vi "Main.vi"() -> ()   [LabVIEW 2020]
uses:
  Typedef/Product Installer.ctl
  Typedef/Custom Action.ctl
  Typedef/Product Installer Definition.ctl
  Typedef/Custom Action Definition.ctl
  Typedef/State.ctl
  Bundle Builder/Bundle Builder.lvclass
  Bundle Builder/Bundle Builder.lvclass/Bundle Builder.ctl
  bd79d48e-615b-41ab-9cb3-2d2f9496b7e1.vi
  Bundle Builder/Read Bundle Definition.vi
  Bundle Builder/Read Bundle Root.vi
  Bundle Builder/Read Product Installers.vi
  Bundle Builder/Read Custom Actions.vi
  Bundle Builder/Read Element of Custom Actions Defnition.vi/bd8829dc-8fc1-4ce8-8fca-fa4916f1d24d.vi
  Bundle Builder/Read Element of Product Installers Definition.vi/92f76918-1563-4c6f-99b4-6a0cba476cd6.vi
  <vilib>/Comparison/Equal/Equal Functor/Equal Functor.lvclass
panel:
  in  "New":bool
  in  "Clear Disk":bool
  in  "Stop Button":bool
  in  "Save":bool
  in  "Tab":T1(tab)
  out "Bundle Root Folder":path
  in  "Bundle Definition":T2
  out "Product Key Unique?":bool
  in  "Product Installers":T3[](array[typedef])
  in  "Product Installer":T4 caption="NI Product Installer / Custom Product Installer"
  in  "Custom Actions":T5[](array[typedef])
  out "Custom Action Key Unique?":bool
  in  "Custom Action":T6
  in  "Open":bool
  in  "Definitions":string(tree)
  # "STS Custom Bundle Builder"
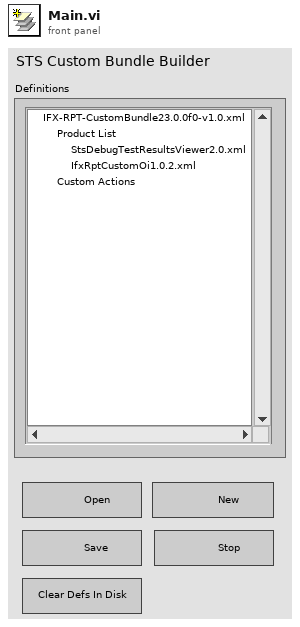
[diagram p1: front panel]
types:
  T1 = enum32{"Default", "Bundle", "Product List", "Product", "Custom Actions", "Custom Action"}
  T2 = cluster{"Key":string, "Display Name":string, "STS Software":string}
  T3 = typedef "Product Installer.ctl" = cluster{"Key":string, "Version":string, "Type":enum16{"NI Installer", "Custom Installer"}}
  T4 = typedef "Product Installer Definition.ctl" = cluster{"Display Name":string, "Install Commands":cluster{"Path":string, "Parameters":string, "Successful Exit Codes":string, "Log Command":cluster{"Flag":string, "File Name":string}}[], "Uninstall Commands":cluster{"Path":string, "Parameters":string, "Successful Exit Codes":string, "Log Command":cluster{"Flag":string, "File Name":string}}[]}
  T5 = typedef "Custom Action.ctl" = cluster{"Key":string, "Timing":string}
  T6 = typedef "Custom Action Definition.ctl" = cluster{"Display Name":string, "Commands":cluster{"Path":string, "Parameters":string, "Successful Exit Codes":string}[]}
  T7 = typedef "State.ctl" = enum16{"Initialize", "Ready", "Open Bundle", "Show Selection Details"}
  T8 = enum8{"Enabled", "Disabled", "Disabled and Grayed Out"}
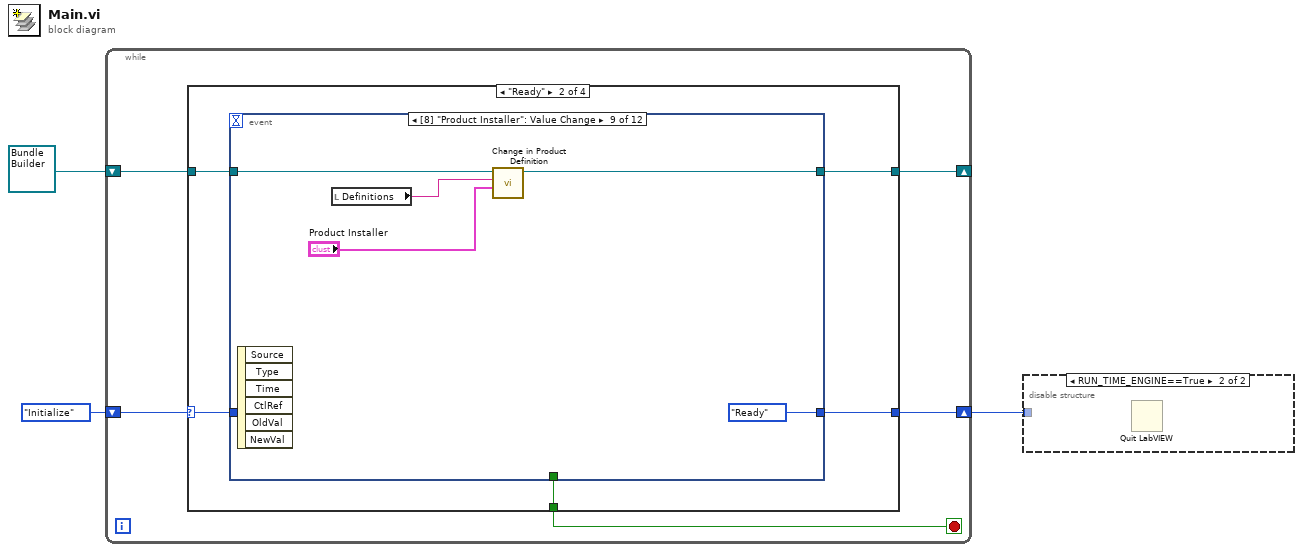
[diagram p0: block diagram]
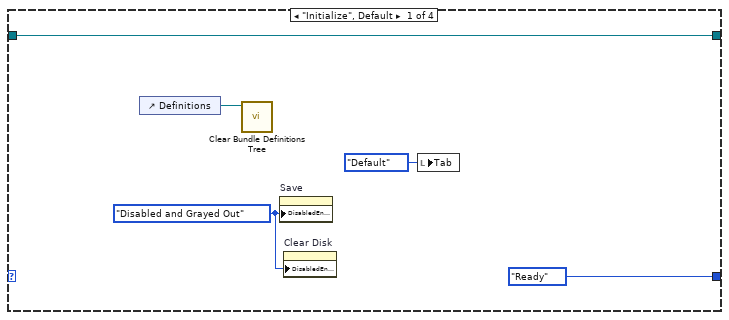
[diagram p3: hidden frame]
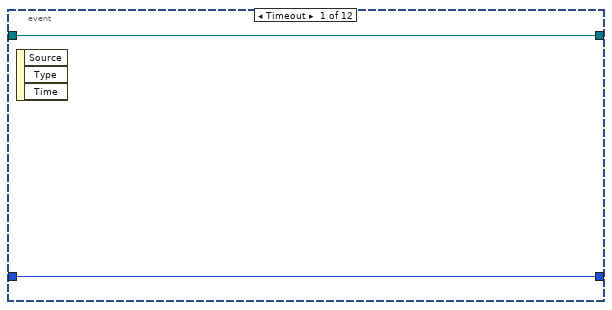
[diagram p4: hidden frame]
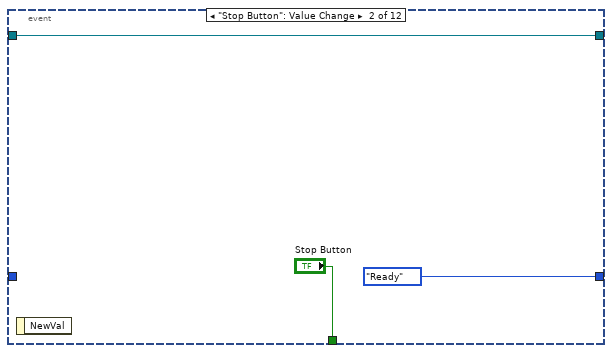
[diagram p5: hidden frame]
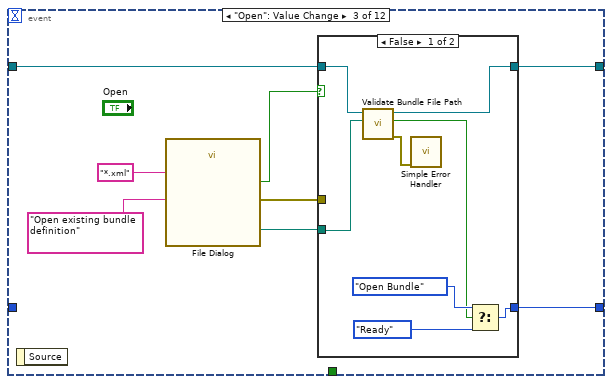
[diagram p6: hidden frame]
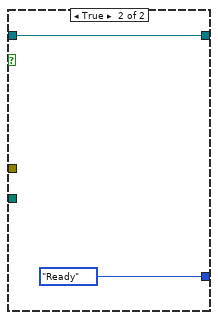
[diagram p7: hidden frame]
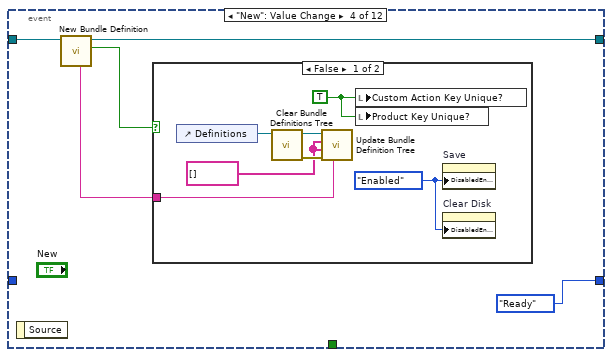
[diagram p8: hidden frame]
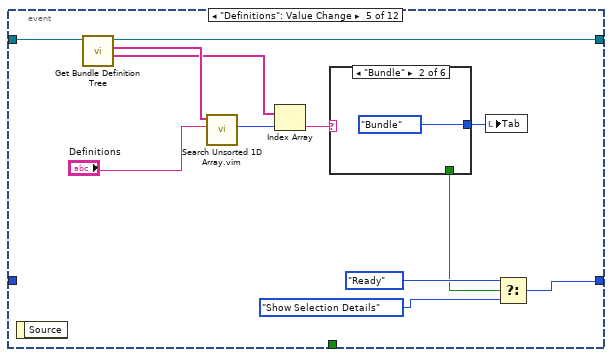
[diagram p10: hidden frame]
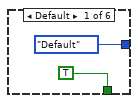
[diagram p11: hidden frame]
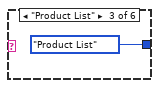
[diagram p12: hidden frame]
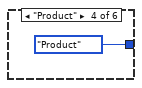
[diagram p13: hidden frame]
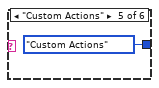
[diagram p14: hidden frame]
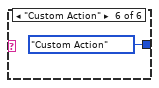
[diagram p15: hidden frame]
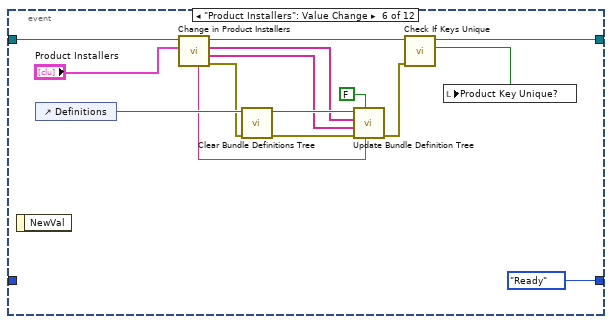
[diagram p16: hidden frame]
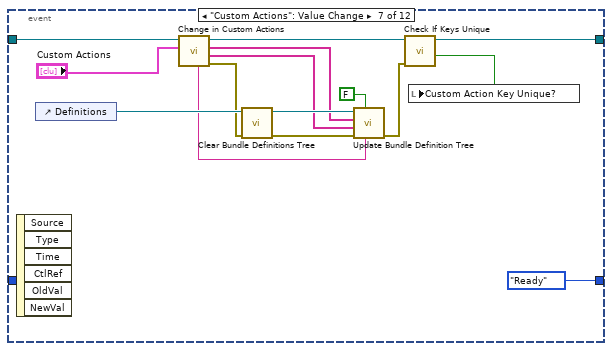
[diagram p17: hidden frame]
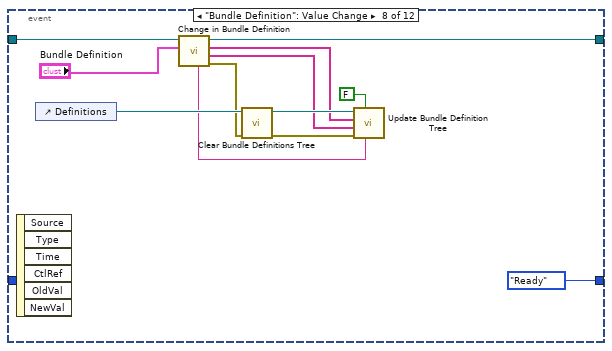
[diagram p18: hidden frame]
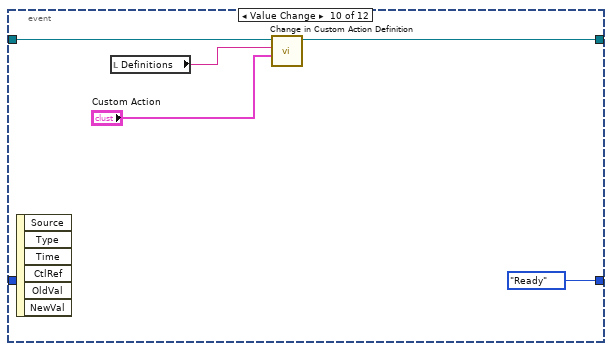
[diagram p19: hidden frame]
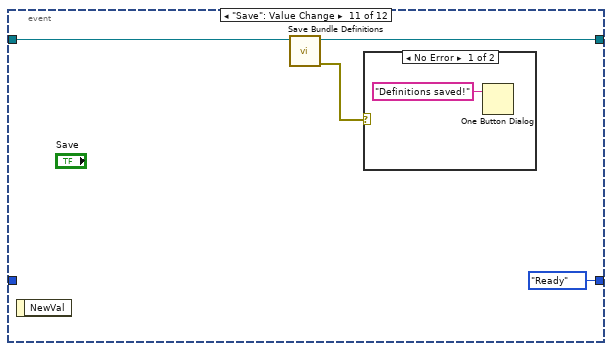
[diagram p20: hidden frame]
diagram:
  n1 = while {
    shift-right: [w4] -> w1
    shift-left: State."Initialize" -> [w8]
    shift-right: [w5] -> _
    shift-left: refnum<class "Bundle Builder.lvclass"> refnum ("Bundle Builder.lvclass") -> [w6]
    stop <- w7 stop-if-true
    n2 = case shown="\"Ready\"" w8 {
      selector: w8 -> [_ w15 _ _]
      tunnel: [_ w18 _ _] -> w7
      tunnel: w6 -> [w12 w17 w155 w160]
      tunnel: [w12 w16 w145 w159] -> w5
      tunnel: [State."Ready" w14 State."Ready" State."Ready"] -> w4
      frame "Initialize", Default {
        w9 = T8."Disabled and Grayed Out" ("Disabled")
        n3 = control-ref of="Definitions"() -> (w13:refnum<vi>)
        n4 = call "Clear Bundle Definitions Tree.vi"("TreeControl in"=w13) -> ()  [unwired: 9 in, 2 out]
        n5 = property on="Save" class="Bool"("DisabledEnum"=w9) -> ()  [unwired: 2 in, 2 out]
        n6 = property on="Clear Disk" class="Bool"("DisabledEnum"=w9) -> ()  [unwired: 2 in, 2 out]
        n7 = local write "Tab"(T1."Default" ("Tab")) -> ()
      }
      frame "Ready" {
        n8 = event shown="[8] \"Product Installer\": Value Change" {
          selector: _ -> [_ _ _ _ _ _ _ _ _ _ _ _]
          dyn-events: _ -> [_ _ _ _ _ _ _ _ _ _ _ _]
          timeout: _ -> [_ _ _ _ _ _ _ _ _ _ _ _]
          tunnel: [_ "Stop Button" _ _ _ _ _ _ _ _ _ _] -> w18
          tunnel: [w19 State."Ready" w28 State."Ready" w56 State."Ready" State."Ready" State."Ready" State."Ready" State."Ready" State."Ready" State."Ready"] -> w14
          tunnel: w17 -> [w20 w21 w31 w46 w65 w87 w102 w114 w119 w124 w128 w135]
          tunnel: [w20 w21 w30 w45 w64 w75 w91 w111 w118 w123 w127 w133] -> w16
          tunnel: w15 -> [w19 _ _ _ _ _ _ _ _ _ _ _]
          event Timeout {
            n9 = event-data() -> ()  [unwired: 1 in, 3 out]
          }
          event "Stop Button": Value Change {
            n10 = event-data() -> ()  [unwired: 1 in, 1 out]
          }
          event "Open": Value Change {
            n11 = event-data() -> ()  [unwired: 1 in, 1 out]
            n12 = call "File Dialog"("prompt"="Open existing bundle definition", "pattern (all files)"="*.xml") -> ("selected path"=w27:path, "cancelled"=w29:bool, "error out"=w24:errorcluster)  [unwired: 10 in, 1 out]
            n13 = case shown="False" w29 {
              tunnel: w31 -> [w37 w41]
              tunnel: [w38 w41] -> w30
              tunnel: [w35 State."Ready"] -> w28
              tunnel: w27 -> [w36 _]
              tunnel: w24 -> [_ _]
              frame False {
                n14 = call "Validate Bundle File Path.vi"("Bundle File Path"=w36, "Bundle Builder in"=w37) -> ("error out"=w32:errorcluster, "Valid?"=w34:bool, "Bundle Builder out"=w38:refnum<class "Bundle Builder.lvclass">)  [unwired: 7 in]
                n15 = call <vilib>:"Simple Error Handler.vi"("error in (no error)"=w32) -> ()  [unwired: 4 in, 5 out]
                n16 = Select(t=State."Open Bundle", s=w34, f=State."Ready") -> (s? t:f=w35:T7)
              }
              frame True {
              }
            }
          }
          event "New": Value Change {
            n17 = event-data() -> ()  [unwired: 1 in, 1 out]
            n18 = call "New Bundle Definition.vi"("Bundle Builder in"=w46) -> ("Cancelled?"=w44:bool, "Bundle Builder out"=w45:refnum<class "Bundle Builder.lvclass">, "Bundle Filename"=w43:string)  [unwired: 7 in, 1 out]
            n19 = case shown="False" w44 {
              tunnel: w43 -> [w49 _]
              frame False {
                w47 = TRUE ("Custom Action Key Unique?")
                w48 = T8."Enabled" ("Disabled")
                w50 = string[] [] ("Product List File Names")
                n20 = control-ref of="Definitions"() -> (w53:refnum<vi>)
                n21 = call "Clear Bundle Definitions Tree.vi"("TreeControl in"=w53) -> ("error out"=w51:errorcluster, "TreeControl out"=w52:refnum<vi>)  [unwired: 9 in]
                n22 = call "Update Bundle Definition Tree.vi"("Bundle Filename"=w49, "error in"=w51, "Custom Actions File Names"=w50, "Product List File Names"=w50, "TreeControl in"=w52) -> ()  [unwired: 5 in, 2 out]
                n23 = local write "Custom Action Key Unique?"(w47) -> ()
                n24 = local write "Product Key Unique?"(w47) -> ()
                n25 = property on="Save" class="Bool"("DisabledEnum"=w48) -> ()  [unwired: 2 in, 2 out]
                n26 = property on="Clear Disk" class="Bool"("DisabledEnum"=w48) -> ()  [unwired: 2 in, 2 out]
              }
              frame True {
              }
            }
          }
          event "Definitions": Value Change {
            n27 = event-data() -> ()  [unwired: 1 in, 1 out]
            n28 = call "Get Bundle Definition Tree.vi"("Bundle Builder in"=w65) -> ("Tree Selection Types"=w61:string[], "Tree Selections"=w63:string[], "Bundle Builder out"=w64:refnum<class "Bundle Builder.lvclass">)  [unwired: 7 in, 1 out]
            n29 = call "Search Unsorted 1D Array.vim"("element"="Definitions", "unsorted 1D array"=w63) -> ("index of element"=w60:i32)  [unwired: 9 in]
            n30 = Index Array(array=w61, index=w60) -> (element=w59:string)
            n31 = case shown="\"Bundle\"" w59 {
              tunnel: [T1."Default" ("Tab") T1."Bundle" ("Tab") T1."Product List" ("Tab") T1."Product" ("Tab") T1."Custom Actions" ("Tab") T1."Custom Action" ("Tab")] -> w58
              tunnel: [TRUE _ _ _ _ _] -> w55
              frame Default {
              }
              frame "Bundle" {
              }
              frame "Product List" {
              }
              frame "Product" {
              }
              frame "Custom Actions" {
              }
              frame "Custom Action" {
              }
            }
            n32 = local write "Tab"(w58) -> ()
            n33 = Select(t=State."Ready", s=w55, f=State."Show Selection Details") -> (s? t:f=w56:T7)
          }
          event "Product Installers": Value Change {
            n34 = event-data() -> ()  [unwired: 1 in, 1 out]
            n35 = control-ref of="Definitions"() -> (w86:refnum<vi>)
            n36 = call "Change in Product Installers.vi"("Product Installers"="Product Installers", "Bundle Builder in"=w87) -> ("error out"=w78:errorcluster, "Custom Actions File Names"=w81:string[], "Product List File Names"=w82:string[], "Bundle Builder out"=w84:refnum<class "Bundle Builder.lvclass">, "Bundle Filename"=w80:string)  [unwired: 5 in]
            n37 = call "Clear Bundle Definitions Tree.vi"("error in"=w78, "TreeControl in"=w86) -> ("error out"=w79:errorcluster, "TreeControl out"=w85:refnum<vi>)  [unwired: 8 in]
            n38 = call "Update Bundle Definition Tree.vi"("Bundle Filename"=w80, "Reset Selection to Root? (T)"=FALSE, "error in"=w79, "Custom Actions File Names"=w81, "Product List File Names"=w82, "TreeControl in"=w85) -> ("error out"=w74:errorcluster)  [unwired: 4 in, 1 out]
            n39 = call "Check If Keys Unique.vi"("error in (no error)"=w74, "Bundle Builder in"=w84) -> ("Product Key Unique?"=w73:bool, "Bundle Builder out"=w75:refnum<class "Bundle Builder.lvclass">)  [unwired: 6 in, 2 out]
            n40 = local write "Product Key Unique?"(w73) -> ()
          }
          event "Custom Actions": Value Change {
            n41 = event-data() -> ()  [unwired: 1 in, 6 out]
            n42 = control-ref of="Definitions"() -> (w101:refnum<vi>)
            n43 = call "Change in Custom Actions.vi"("Custom Actions"="Custom Actions", "Bundle Builder in"=w102) -> ("error out"=w94:errorcluster, "Custom Actions File Names"=w97:string[], "Product List File Names"=w98:string[], "Bundle Builder out"=w99:refnum<class "Bundle Builder.lvclass">, "Bundle Filename"=w96:string)  [unwired: 5 in]
            n44 = call "Clear Bundle Definitions Tree.vi"("error in"=w94, "TreeControl in"=w101) -> ("error out"=w95:errorcluster, "TreeControl out"=w100:refnum<vi>)  [unwired: 8 in]
            n45 = call "Update Bundle Definition Tree.vi"("Bundle Filename"=w96, "Reset Selection to Root? (T)"=FALSE, "error in"=w95, "Custom Actions File Names"=w97, "Product List File Names"=w98, "TreeControl in"=w100) -> ("error out"=w90:errorcluster)  [unwired: 4 in, 1 out]
            n46 = call "Check If Keys Unique.vi"("error in (no error)"=w90, "Bundle Builder in"=w99) -> ("Custom Action Key Unique?"=w88:bool, "Bundle Builder out"=w91:refnum<class "Bundle Builder.lvclass">)  [unwired: 6 in, 2 out]
            n47 = local write "Custom Action Key Unique?"(w88) -> ()
          }
          event "Bundle Definition": Value Change {
            n48 = event-data() -> ()  [unwired: 1 in, 6 out]
            n49 = control-ref of="Definitions"() -> (w113:refnum<vi>)
            n50 = call "Change in Bundle Definition.vi"("Bundle Definition"="Bundle Definition", "Bundle Builder in"=w114) -> ("error out"=w106:errorcluster, "Custom Actions File Names"=w109:string[], "Product List File Names"=w110:string[], "Bundle Builder out"=w111:refnum<class "Bundle Builder.lvclass">, "Bundle Filename"=w108:string)  [unwired: 5 in]
            n51 = call "Clear Bundle Definitions Tree.vi"("error in"=w106, "TreeControl in"=w113) -> ("error out"=w107:errorcluster, "TreeControl out"=w112:refnum<vi>)  [unwired: 8 in]
            n52 = call "Update Bundle Definition Tree.vi"("Bundle Filename"=w108, "Reset Selection to Root? (T)"=FALSE, "error in"=w107, "Custom Actions File Names"=w109, "Product List File Names"=w110, "TreeControl in"=w112) -> ()  [unwired: 4 in, 2 out]
          }
          event Value Change {
            n53 = event-data() -> ()  [unwired: 1 in, 6 out]
            n54 = local read "Definitions"() -> (w116:string)
            n55 = call "Change in Product Definition.vi"("Product Installer"="Product Installer", "Selected Product File Name"=w116, "Bundle Builder in"=w119) -> ("Bundle Builder out"=w118:refnum<class "Bundle Builder.lvclass">)  [unwired: 7 in, 1 out]
          }
          event Value Change {
            n56 = event-data() -> ()  [unwired: 1 in, 6 out]
            n57 = local read "Definitions"() -> (w121:string)
            n58 = call "Change in Custom Action Definition.vi"("Custom Action"="Custom Action", "Selected Custom Action File Name"=w121, "Bundle Builder in"=w124) -> ("Bundle Builder out"=w123:refnum<class "Bundle Builder.lvclass">)  [unwired: 7 in, 1 out]
          }
          event "Save": Value Change {
            n59 = event-data() -> ()  [unwired: 1 in, 1 out]
            n60 = call "Save Bundle Definitions.vi"("Bundle Builder in"=w128) -> ("error out"=w126:errorcluster, "Bundle Builder out"=w127:refnum<class "Bundle Builder.lvclass">)  [unwired: 9 in]
            n61 = case shown="No Error" w126 {
              selector: w126 -> [_ w130]
              frame No Error {
                n62 = One Button Dialog(message="Definitions saved!") -> ()  [unwired: 1 in, 1 out]
              }
              frame Error {
                n63 = call <vilib>:"Simple Error Handler.vi"("error in (no error)"=w130) -> ()  [unwired: 4 in, 5 out]
              }
            }
          }
          event "Clear Disk": Value Change {
            n64 = event-data() -> ()  [unwired: 1 in, 2 out]
            n65 = Two Button Dialog(message="Are you sure want to clear all the definition files (xml) in the Bundle Definitions, NI Product Definitions and Custom Definitions folder?") -> (T button?=w132:bool)  [unwired: 2 in]
            n66 = case shown="True" w132 {
              tunnel: w135 -> [w136 w139]
              tunnel: [w136 w138] -> w133
              frame False {
              }
              frame True {
                n67 = call "Clear All Definitions in Disk.vi"("Bundle Builder in"=w139) -> ("error out"=w137:errorcluster, "Bundle Builder out"=w138:refnum<class "Bundle Builder.lvclass">)  [unwired: 9 in]
                n68 = call <vilib>:"Simple Error Handler.vi"("error in (no error)"=w137) -> ()  [unwired: 4 in, 5 out]
              }
            }
          }
        }
      }
      frame "Open Bundle" {
        w140 = T8."Enabled" ("Disabled")
        n69 = control-ref of="Definitions"() -> (w153:refnum<vi>)
        n70 = call "Open Bundle.vi"("Bundle Builder in"=w155) -> ("error out"=w147:errorcluster, "Custom Actions File Names"=w151:string[], "Product List File Names"=w152:string[], "Bundle Builder out"=w154:refnum<class "Bundle Builder.lvclass">, "Bundle Filename"=w150:string)  [unwired: 6 in]
        n71 = call "Clear Bundle Definitions Tree.vi"("error in"=w147, "TreeControl in"=w153) -> ("error out"=w146:errorcluster, "TreeControl out"=w148:refnum<vi>)  [unwired: 8 in]
        n72 = call "Update Bundle Definition Tree.vi"("Bundle Filename"=w150, "error in"=w146, "Custom Actions File Names"=w151, "Product List File Names"=w152, "TreeControl in"=w148) -> ("error out"=w144:errorcluster)  [unwired: 5 in, 1 out]
        n73 = call "Check If Keys Unique.vi"("error in (no error)"=w144, "Bundle Builder in"=w154) -> ("error out"=w141:errorcluster, "Custom Action Key Unique?"=→"Custom Action Key Unique?":bool, "Product Key Unique?"=→"Product Key Unique?":bool, "Bundle Builder out"=w145:refnum<class "Bundle Builder.lvclass">)  [unwired: 6 in]
        n74 = call <vilib>:"Simple Error Handler.vi"("error in (no error)"=w141) -> ()  [unwired: 4 in, 5 out]
        n75 = property on="Save" class="Bool"(error in=w141, "DisabledEnum"=w140) -> ()  [unwired: 1 in, 2 out]
        n76 = property on="Clear Disk" class="Bool"(error in=w141, "DisabledEnum"=w140) -> ()  [unwired: 1 in, 2 out]
      }
      frame "Show Selection Details" {
        n77 = local read "Definitions"() -> (w157:string)
        n78 = case shown="\"Bundle\"" "Tab" {
          tunnel: w160 -> [w161 w165 w168 w171 w175 w179]
          tunnel: [w161 w164 w167 w170 w174 w178] -> w159
          tunnel: w157 -> [_ _ _ _ w172 w176]
          frame Default {
          }
          frame "Bundle" {
            n79 = property on="Property Node" class="Bundle Builder.lvclass"(reference=w165) -> (reference out=w164:refnum<class "Bundle Builder.lvclass">, "Bundle Definition"=w163:T2, "Bundle Root"=→"Bundle Root Folder":path)  [unwired: 1 in, 1 out]
            n80 = local write "Bundle Definition"(w163) -> ()
          }
          frame "Product List" {
            n81 = property on="Property Node" class="Bundle Builder.lvclass"(reference=w168) -> (reference out=w167:refnum<class "Bundle Builder.lvclass">, "Product Installers"=w166:T3[])  [unwired: 1 in, 1 out]
            n82 = local write "Product Installers"(w166) -> ()
          }
          frame "Custom Actions" {
            n83 = property on="Property Node" class="Bundle Builder.lvclass"(reference=w171) -> (reference out=w170:refnum<class "Bundle Builder.lvclass">, "Custom Actions"=w169:T5[])  [unwired: 1 in, 1 out]
            n84 = local write "Custom Actions"(w169) -> ()
          }
          frame "Custom Action" {
            n85 = call "Read Element of Custom Actions Defnition.vi"("Selected Custom Action File Name"=w172, "Bundle Builder in"=w175) -> ("Custom Actions"=w173:T6, "Bundle Builder out"=w174:refnum<class "Bundle Builder.lvclass">)  [unwired: 7 in, 1 out]
            n86 = local write "Custom Action"(w173) -> ()
          }
          frame "Product" {
            n87 = call "Read Element of Product Installers Definition.vi"("Selected Product File Name"=w176, "Bundle Builder in"=w179) -> ("Product Installer"=w177:T4, "Bundle Builder out"=w178:refnum<class "Bundle Builder.lvclass">)  [unwired: 7 in, 1 out]
            n88 = local write "Product Installer"(w177) -> ()
          }
        }
      }
    }
  }
  n89 = disable-structure "Conditional Disable Structure" shown="RUN_TIME_ENGINE==True" {
    disable-tunnel: w1 -> [_ _]
    frame condition #0 (active) {
    }
    frame condition #1 {
      n90 = Quit LabVIEW() -> ()  [unwired: 1 in]
    }
  }
